vi "SVT AC Synchronous Motor.vi"(0 "nominal speed [RPM]":dbl=1800.0, 1 "desired units":u16(ring) items=["Hz", "Order"], 5 "number of poles":u32=4, 7 "coils per pole":u32=50, 9 "line frequency [Hz]":dbl=60.0, 11 "error in (no error)":errorcluster) -> (3 "number of stator coils":u32=200, 4 "coil pass frequency":dbl=6000.0, 15 "error out":errorcluster)   [LabVIEW 2017, in "SoundVib_MachineCharacteristic.lvlib"]
doc: "Calculates characteristic frequencies or orders of motors. You must manually select the polymorphic instance you want to use."
uses:
  <vilib>/addons/Sound and Vibration/svt_Machine Characteristic/SoundVib_MachineCharacteristic.lvlib
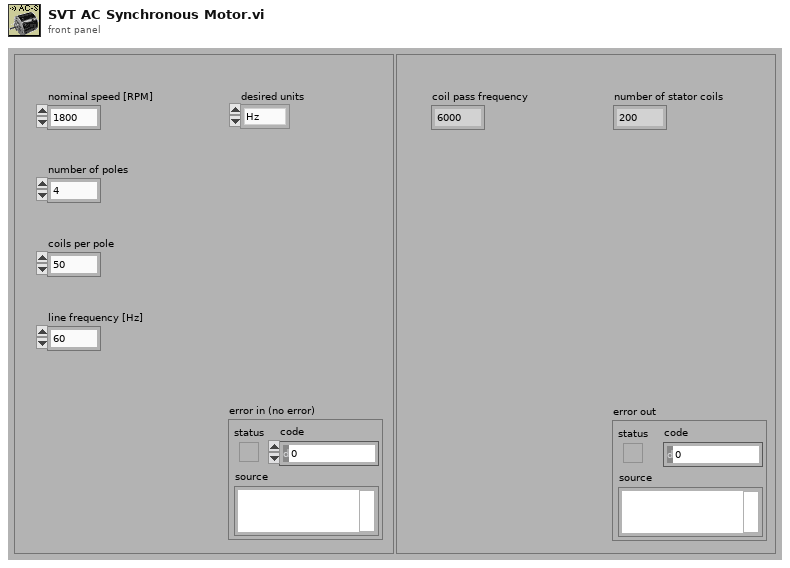
[diagram p1: front panel]
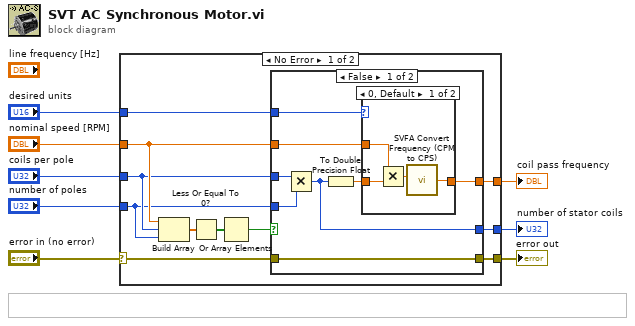
[diagram p0: block diagram]
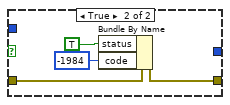
[diagram p3: hidden frame]
diagram:
  n1 = case shown="No Error" "error in (no error)" {
    selector: "error in (no error)" -> [w16 w37]
    tunnel: [w15 w37] -> w7
    tunnel: "nominal speed [RPM]" -> [w14 _]
    tunnel: "desired units" -> [w19 _]
    tunnel: "coils per pole" -> [w13 _]
    tunnel: "number of poles" -> [w12 _]
    tunnel: [w18 _] -> w2
    tunnel: [w17 _] -> w1
    frame No Error {
      n2 = Build Array(w14, w13, w12) -> (w11:dbl[])
      n3 = Less Or Equal To 0?(x=w11) -> (x <= 0?=w10:bool[])
      n4 = Or Array Elements(Boolean array=w10) -> (logical OR=w9:bool)
      n5 = case shown="False" w9 {
        tunnel: w19 -> [w27 _]
        tunnel: w13 -> [w26 _]
        tunnel: w12 -> [w25 _]
        tunnel: w14 -> [w24 _]
        tunnel: [w22 _] -> w18
        tunnel: [w23 _] -> w17
        tunnel: w16 -> [w20 w34]
        tunnel: [w20 w33] -> w15
        frame False {
          n6 = Multiply(x=w26, y=w25) -> (x*y=w22:u32)
          n7 = To Double Precision Float(number=w22) -> (double precision float=w21:dbl)
          n8 = case shown="0, Default" w27 {
            tunnel: w21 -> [w31 w32]
            tunnel: w24 -> [w30 _]
            tunnel: [w28 w32] -> w23
            frame 0, Default {
              n9 = Multiply(x=w30, y=w31) -> (x*y=w29:dbl)
              n10 = call <vilib>:"SVFA Convert Frequency (CPM to CPS).vi"("nominal speed [RPM]"=w29) -> ("frequency [Hz]"=w28:dbl)  [unwired: 5 in]
            }
            frame 1 {
            }
          }
        }
        frame True {
          n11 = Bundle By Name(cluster=w34, "status"=TRUE, "code"=-1984) -> (w33:errorcluster)
        }
      }
    }
    frame Error {
    }
  }
  "coil pass frequency" <- w1
  "number of stator coils" <- w2
  "error out" <- w7
